vi "High-Level Write to Text File - N-Channel.vi"() -> ()   [LabVIEW 2019]
uses:
  <vilib>/DAQmx/read.llb/DAQmx Read (Analog 2D DBL NChan NSamp).vi
  <vilib>/DAQmx/create/channels.llb/DAQmx Create Channel (AI-Voltage-Basic).vi
  <vilib>/DAQmx/configure/timing.llb/DAQmx Timing (Sample Clock).vi
  <vilib>/DAQmx/miscellaneous.llb/DAQmx Fill In Error Info.vi
  <vilib>/Utility/file.llb/Write Delimited Spreadsheet (string).vi
  <vilib>/Utility/file.llb/Write Delimited Spreadsheet (DBL).vi
  <resource>/objmgr/daqmx.rc
panel:
  out "Waveform Graph":dbl[][](graph)
  in  "Data log filepath":path
  in  "minimum value":dbl=-5.0
  in  "maximum value":dbl=5.0
  in  "Number of Samples":i32=100
  in  "Desired Sample Rate (Hz)":dbl=1000.0
  in  "Physical Channel":tag="PCI-6221/ai0:3"
  out "Actual Sample Rate (Hz)":dbl
  # "Measurement Range"
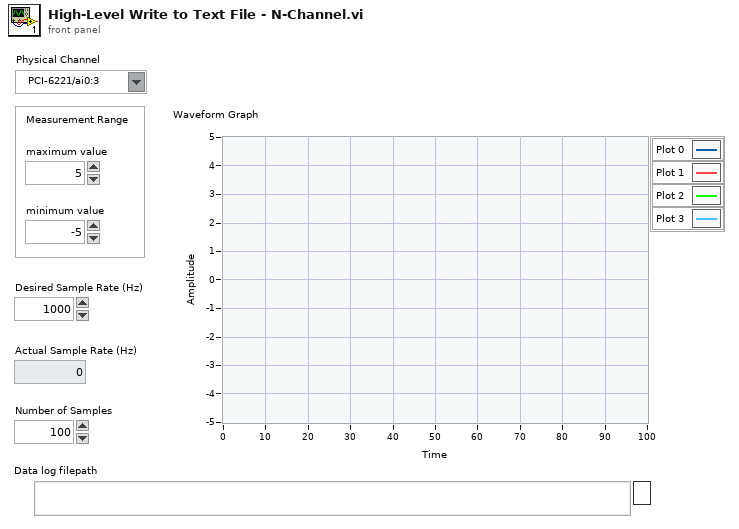
[diagram p1: front panel]
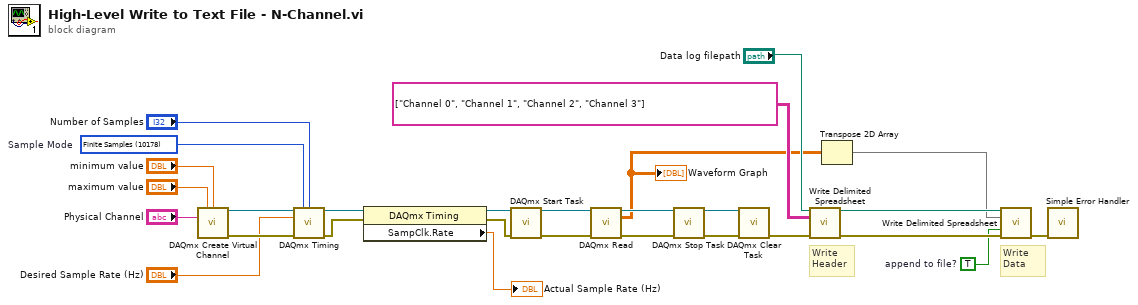
[diagram p0: block diagram]
diagram:
  w14 = 10178 items=["Finite Samples"=10178, "Continuous Samples"=10123, "Hardware Timed Single Point"=12522]  # Sample Mode
  w16 = TRUE  # append to file?
  # "Write Data"
  # "Write Header"
  n1 = call-poly <vilib>:"DAQmx Create Virtual Channel.vi"("maximum value"="maximum value", "minimum value"="minimum value", "physical channels"="Physical Channel") -> ("task out"=w28:refnum<k21>, "error out"=w27:errorcluster)  [unwired: 11 in]
  n2 = call-poly <vilib>:"DAQmx Timing.vi"("task/channels in"=w28, "sample mode"=w14, "samples per channel"="Number of Samples", "rate"="Desired Sample Rate (Hz)", "error in"=w27) -> ("task out"=w26:refnum<k21>, "error out"=w25:errorcluster)  [unwired: 9 in]
  n3 = property class="DAQmx Timing"(reference=w26, error in=w25) -> (reference out=w24:refnum<k21>, error out=w23:errorcluster, "SampClk.Rate"=→"Actual Sample Rate (Hz)":dbl)
  n4 = call <vilib>:"DAQmx Start Task.vi"("task/channels in"=w24, "error in"=w23) -> ("task out"=w22:refnum<k21>, "error out"=w21:errorcluster)  [unwired: 12 in]
  n5 = call-poly <vilib>:"DAQmx Read.vi"("task/channels in"=w22, "error in"=w21) -> ("task out"=w13:refnum<k21>, "data"=w1:dbl[][], "error out"=w12:errorcluster)  [unwired: 11 in]
  "Waveform Graph" <- w1
  n6 = call <vilib>:"DAQmx Stop Task.vi"("task/channels in"=w13, "error in"=w12) -> ("task out"=w11:refnum<k21>, "error out"=w10:errorcluster)  [unwired: 12 in]
  n7 = call <vilib>:"DAQmx Clear Task.vi"("task in"=w11, "error in"=w10) -> ("error out"=w19:errorcluster)  [unwired: 13 in]
  n8 = call-poly <vilib>:"Write Delimited Spreadsheet.vi"("file path (dialog if empty)"="Data log filepath", "2D data"=string[][] [["Channel 0", "Channel 1", "Channel 2", "Channel 3"]], "error in (no error)"=w19) -> ("new file path (Not A Path if cancelled)"=w18:path, "error out"=w17:errorcluster)  [unwired: 11 in]
  n9 = Transpose 2D Array(2D array=w1) -> (transposed array=w9:dbl[][])
  n10 = call-poly <vilib>:"Write Delimited Spreadsheet.vi"("file path (dialog if empty)"=w18, "2D data"=w9, "append to file? (new file:F)"=w16, "error in (no error)"=w17) -> ("error out"=w15:errorcluster)  [unwired: 10 in, 1 out]
  n11 = call <vilib>:"Simple Error Handler.vi"("error in (no error)"=w15) -> ()  [unwired: 4 in, 5 out]
